vi "DSF.Engine.Transceiver Thread.Launch.vi"(8 "error in (no error)":errorcluster, 9 "Thread ID Pool":refnum<class "DSF.Engine.Pool.ID.lvclass">, 10 "Thread Parameters":refnum<class "Thread Parameters.lvclass">, 11 "Transceiver Thread in":refnum<class "DSF.Engine.Transceiver Thread.lvclass">) -> (0 "error out":errorcluster, 3 "Transceiver Thread out":refnum<class "DSF.Engine.Transceiver Thread.lvclass">)   [LabVIEW 2017, in "DSF.Engine.lvlib" / "DSF.Engine.Transceiver Thread.lvclass"]
uses:
  DSF.Engine.Transceiver Thread.lvclass
  Thread Parameters/Thread Parameters.lvclass
  Interface/DSF.Engine.Interface.Transceiver.lvclass
  Thread Pool/DSF.Engine.Pool.ID.lvclass
  DSF.Engine.Transceiver Thread.lvclass/DSF.Engine.Transceiver Thread.ctl
  DSF.Engine.Transceiver Thread.Main.vi
panel:
  out "Interface":refnum<class "DSF.Engine.Interface.Transceiver.lvclass">
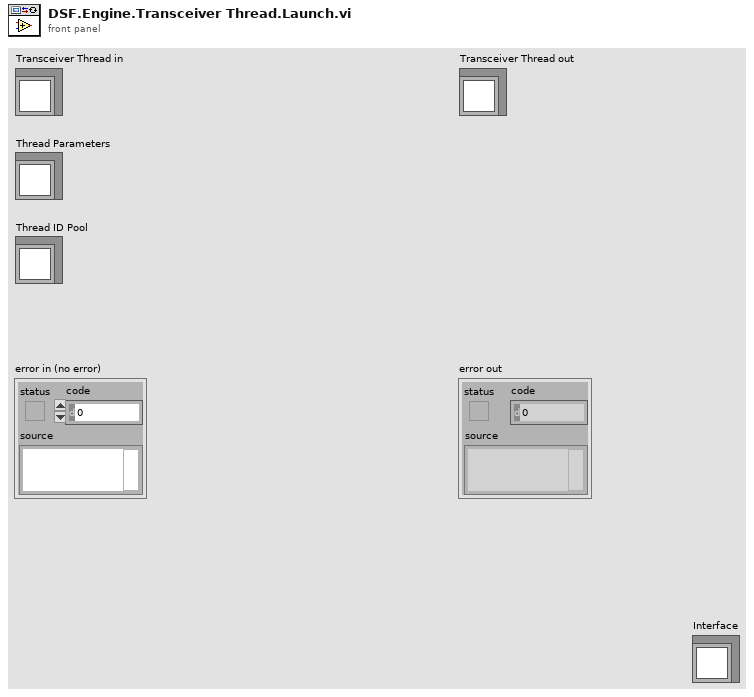
[diagram p1: front panel]
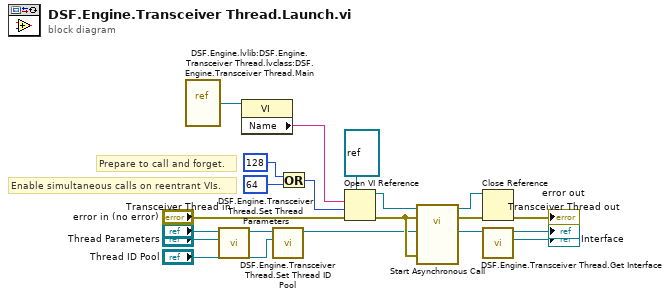
[diagram p0: block diagram]
diagram:
  # "Prepare to call and forget."
  # "Enable simultaneous calls on reentrant VIs."
  n1 = vi-ref "DSF.Engine.lvlib:DSF.Engine.Transceiver Thread.lvclass:DSF.Engine.Transceiver Thread.Main.vi"() -> (w2:refnum<vi>)
  n2 = call "DSF.Engine.Transceiver Thread.Set Thread Parameters.vi"("Thread Parameters"="Thread Parameters", "Transceiver Thread in"="Transceiver Thread in") -> ("Transceiver Thread out"=w5:refnum<class "DSF.Engine.Transceiver Thread.lvclass">)  [unwired: 9 in]
  n3 = property class="VI"(reference=w2) -> ("Name"=w1:string)  [unwired: 1 in, 2 out]
  n4 = call "DSF.Engine.Transceiver Thread.Set Thread ID Pool.vi"("Thread ID Pool"="Thread ID Pool", "Transceiver Thread in"=w5) -> ("Transceiver Thread out"=w4:refnum<class "DSF.Engine.Transceiver Thread.lvclass">)  [unwired: 9 in]
  n5 = Or(x=128 ("options"), y=64 ("options")) -> (x .or. y?=w12:i32)
  n6 = Open VI Reference(type specifier VI Refnum (for type only)=refnum<vi> refnum, vi path=w1, options=w12, error in (no error)="error in (no error)") -> (vi reference=w17:refnum<vi>, error out=w18:errorcluster)  [unwired: 2 in]
  n7 = call-by-ref "Start Asynchronous Call"(reference=w17, error in=w18, 8:"error in (no error)"=w18, "Transceiver Thread in"=w4) -> (reference out=w15:refnum<vi>, error out=w16:errorcluster)  [unwired: 8 in, 2 out]
  n8 = Close Reference(reference=w15, error in (no error)=w16) -> (error out=→"error out":errorcluster)
  n9 = call "DSF.Engine.Transceiver Thread.Get Interface.vi"("Transceiver Thread in"=w4) -> ("Interface"=→"Interface":refnum<class "DSF.Engine.Interface.Transceiver.lvclass">, "Transceiver Thread out"=→"Transceiver Thread out":refnum<class "DSF.Engine.Transceiver Thread.lvclass">)  [unwired: 9 in]
